vi "formatCfmToString.vi"(8 "error in (no error)":errorcluster, 9 "CFM 1":dynamicdata(waveform), 10 "CFM 2":dynamicdata(waveform), 11 "CFM 3":dynamicdata(waveform)) -> (0 "error out":errorcluster, 3 "String":string)   [LabVIEW 2019]
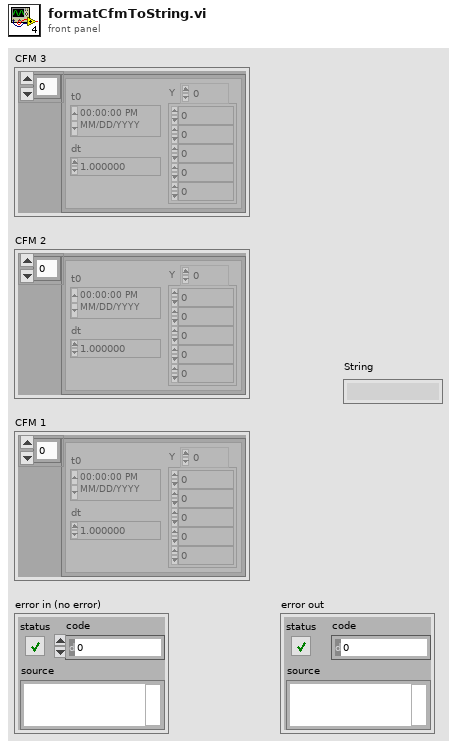
[diagram p1: front panel]
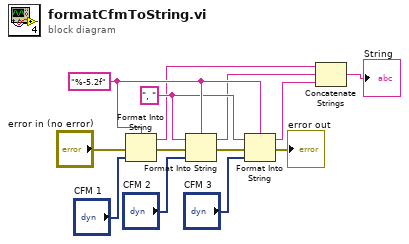
[diagram p0: block diagram]
diagram:
  w5 = ", "
  w13 = "%-5.2f" ("format string")
  n1 = Format Into String(format string=w13, error in="error in (no error)", "CFM 1") -> (resulting string=w4:string, error out=w11:errorcluster)  [unwired: 1 in]
  n2 = Format Into String(format string=w13, initial string=w5, error in=w11, "CFM 2") -> (resulting string=w3:string, error out=w12:errorcluster)
  n3 = Format Into String(format string=w13, initial string=w5, error in=w12, "CFM 3") -> (resulting string=w2:string, error out=→"error out":errorcluster)
  n4 = Concatenate Strings(w4, w3, w2) -> (→"String":string)
